vi "SPARK Configure Signal Period.vi"(8 "error in":errorcluster, 9 "Period (ms)":u32, 10 "Signal":T1, 11 "MotorControlDeviceRef":T2={"DeviceStatus"={"status"=FALSE, "code"=0, "source"=""}, "Type"=enum."PWM", "PWM"={"PWM Channel"=enum."Invalid", "DeadBand"={"Name"="", "maxPositivePwm"=0, "minPositivePwm"=0, "centerPwm"=0, "maxNegativePwm"=0, "minNegativePwm"=0, "angularRange"=0}}, "CAN"={"Device Number"=0, "SetOutput VI Ref"=variant(refnum<vi> refnum), "GetOutput VI Ref"=variant(refnum<vi> refnum), "Enable VI Ref"=variant(refnum<vi> refnum), "Disable VI Ref"=variant(refnum<vi> refnum), "Data"=variant}, "Invert"=FALSE, "DIO PWM"={"PWM \"Enable\" Channel"=enum."Invalid", "DIOChannel"=enum."Invalid", "PWM Rate"=0.0}}) -> (0 "error out":errorcluster, 3 "MotorControlDeviceRef":T2={"DeviceStatus"={"status"=FALSE, "code"=0, "source"=""}, "Type"=enum."PWM", "PWM"={"PWM Channel"=enum."Invalid", "DeadBand"={"Name"="", "maxPositivePwm"=0, "minPositivePwm"=0, "centerPwm"=0, "maxNegativePwm"=0, "minNegativePwm"=0, "angularRange"=0}}, "CAN"={"Device Number"=0, "SetOutput VI Ref"=variant(refnum<vi> refnum), "GetOutput VI Ref"=variant(refnum<vi> refnum), "Enable VI Ref"=variant(refnum<vi> refnum), "Disable VI Ref"=variant(refnum<vi> refnum), "Data"=variant}, "Invert"=FALSE, "DIO PWM"={"PWM \"Enable\" Channel"=enum."Invalid", "DIOChannel"=enum."Invalid", "PWM Rate"=0.0}})   [LabVIEW 2023]
doc: "Configure the period of a signal. This will be the rate at which the SPARK will send the periodic status that contains the specificed signal."
uses:
  <vilib>/Rock Robotics/WPI/MotorControl/WPI_MotorControlDeviceRef.ctl
  <vilib>/Rock Robotics/WPI/MotorControl/WPI_MotorControlType.ctl
  <vilib>/Rock Robotics/SystemInterfaces/DIO/FPGA_DIOPWMChannel.ctl
  <vilib>/Rock Robotics/WPI/PWM/WPI_PWMDeadband.ctl
  <vilib>/Rock Robotics/SystemInterfaces/DIO/FPGA_DIOChannel.ctl
  Typedef/SPARK Signal.ctl
  Typedef/SPARK Parameter ID.ctl
  Typedef/Spark MAX Variant Data.ctl
  Typedef/SPARK Model.ctl
  Private/SPARK/SPARK Set Parameter Uint32.vi
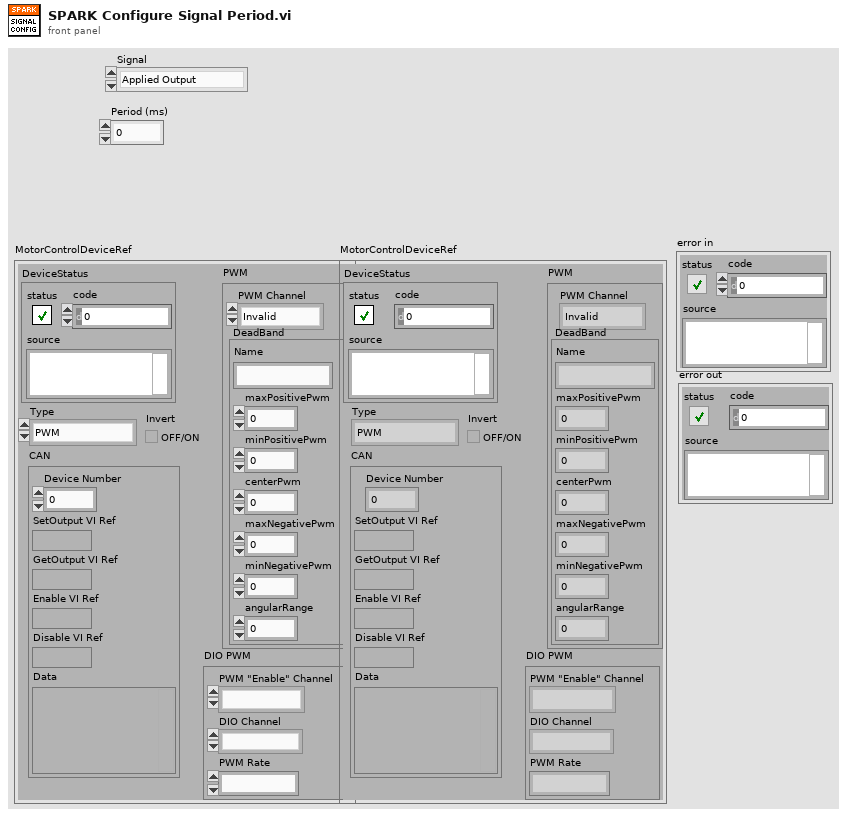
[diagram p1: front panel]
types:
  T1 = typedef "SPARK Signal.ctl" = enum16{"Applied Output", "Bus Voltage", "Output Current", "Motor Temperature", "Limits", "Faults", "Warnings", "Primary Encoder Velocity", "Primary Encoder Position", "Analog Voltage", "Analog Velocity", "Analog Position", "Alt/Ext Encoder Velocity", "Alt/Ext Encoder Position", "Absolute Encoder Velocity", "Absolute Encoder Position", "I Accumulation", "At Setpoint", "Setpoint", "Selected Closed Loop Slot", "MAXMotion Position Setpoint", "MAXMotion Velocity Setpoint"}
  T2 = typedef "WPI_MotorControlDeviceRef.ctl" = cluster{"DeviceStatus":errorcluster, "Type":T3, "PWM":cluster{"PWM Channel":T4, "DeadBand":T5}, "CAN":cluster{"Device Number":u8, "SetOutput VI Ref":variant, "GetOutput VI Ref":variant, "Enable VI Ref":variant, "Disable VI Ref":variant, "Data":variant}, "Invert":bool, "DIO PWM":cluster{"PWM \"Enable\" Channel":T4, "DIOChannel":T6, "PWM Rate":dbl}}
  T3 = typedef "WPI_MotorControlType.ctl" = enum16{"PWM", "CAN", "DIO PWM"}
  T4 = typedef "FPGA_DIOPWMChannel.ctl" = enum8{"PWM 0", "PWM 1", "PWM 2", "PWM 3", "PWM 4", "PWM 5", "PWM 6", "PWM 7", "PWM 8", "PWM 9", "PWM MXP 0", "PWM MXP 1", "PWM MXP 2", "PWM MXP 3", "PWM MXP 4", "PWM MXP 5", "PWM MXP 6", "PWM MXP 7", "PWM MXP 8", "PWM MXP 9", "Invalid"}
  T5 = typedef "WPI_PWMDeadband.ctl" = cluster{"Name":string, "maxPositivePwm":i32, "minPositivePwm":i32, "centerPwm":i32, "maxNegativePwm":i32, "minNegativePwm":i32, "angularRange":u16}
  T6 = typedef "FPGA_DIOChannel.ctl" = enum8{"DIO 0", "DIO 1", "DIO 2", "DIO 3", "DIO 4", "DIO 5", "DIO 6", "DIO 7", "DIO 8", "DIO 9", "DIO MXP 0", "DIO MXP 1", "DIO MXP 2", "DIO MXP 3", "DIO MXP 4", "DIO MXP 5", "DIO MXP 6", "DIO MXP 7", "DIO MXP 8", "DIO MXP 9", "DIO MXP 10", "DIO MXP 11", "DIO MXP 12", "DIO MXP 13", "DIO MXP 14", "DIO MXP 15", "SPI Port CS1", "SPI Port CS2", "SPI Port CS3", "SPI Port MISO", "SPI Port MOSI", "Invalid"}
  T7 = typedef "SPARK Parameter ID.ctl" = enum16{"kCanID", "kInputMode", "kMotorType", "kCommAdvance", "kSensorType", "kCtrlType", "kIdleMode", "kInputDeadband", "kLegacyFeedbackSensorPID0", "kClosedLoopControlSensor", "kPolePairs", "kCurrentChop", "kCurrentChopCycles", "kP_0", "kI_0", "kD_0", "kV_0", "kIZone_0", "kDFilter_0", "kOutputMin_0", "kOutputMax_0", "kP_1", "kI_1", "kD_1", "kV_1", "kIZone_1", "kDFilter_1", "kOutputMin_1", "kOutputMax_1", "kP_2", "kI_2", "kD_2", "kV_2", "kIZone_2", "kDFilter_2", "kOutputMin_2", "kOutputMax_2", "kP_3", "kI_3", "kD_3", "kV_3", "kIZone_3", "kDFilter_3", "kOutputMin_3", "kOutputMax_3", "kInverted", "kOutputRatio", "kSerialNumberLow", "kSerialNumberMid", "kSerialNumberHigh", "kLimitSwitchFwdPolarity", "kLimitSwitchRevPolarity", "kHardLimitFwdEn", "kHardLimitRevEn", "kSoftLimitFwdEn", "kSoftLimitRevEn", "kRampRate", "kFollowerID", "kFollowerConfig", "kSmartCurrentStallLimit", "kSmartCurrentFreeLimit", "kSmartCurrentConfig", "kSmartCurrentReserved", "kMotorKv", "kMotorR", "kMotorL", "kMotorRsvd1", "kMotorRsvd2", "kMotorRsvd3", "kEncoderCountsPerRev", "kEncoderAverageDepth", "kEncoderSampleDelta", "kEncoderInverted", "kEncoderRsvd1", "kClosedLoopVoltageMode", "kCompensatedNominalVoltage", "kSmartMotionMaxVelocity_0", "kSmartMotionMaxAccel_0", "kSmartMotionMinVelOutput_0", "kSmartMotionAllowedClosedLoopError_0", "kSmartMotionAccelStrategy_0", "kSmartMotionMaxVelocity_1", "kSmartMotionMaxAccel_1", "kSmartMotionMinVelOutput_1", "kSmartMotionAllowedClosedLoopError_1", "kSmartMotionAccelStrategy_1", "kSmartMotionMaxVelocity_2", "kSmartMotionMaxAccel_2", "kSmartMotionMinVelOutput_2", "kSmartMotionAllowedClosedLoopError_2", "kSmartMotionAccelStrategy_2", "kSmartMotionMaxVelocity_3", "kSmartMotionMaxAccel_3", "kSmartMotionMinVelOutput_3", "kSmartMotionAllowedClosedLoopError_3", "kSmartMotionAccelStrategy_3", "kIMaxAccum_0", "kAllowedClosedLoopError_0", "kSlot3Placeholder2_0", "kSlot3Placeholder3_0", "kIMaxAccum_1", "kAllowedClosedLoopError_1", "kSlot3Placeholder2_1", "kSlot3Placeholder3_1", "kIMaxAccum_2", "kAllowedClosedLoopError_2", "kSlot3Placeholder2_2", "kSlot3Placeholder3_2", "kIMaxAccum_3", "kAllowedClosedLoopError_3", "kSlot3Placeholder2_3", "kSlot3Placeholder3_3", "kPositionConversionFactor", "kVelocityConversionFactor", "kClosedLoopRampRate", "kSoftLimitFwd", "kSoftLimitRev", "kSoftLimitRsvd0", "kSoftLimitRsvd1", "kAnalogPositionConversion", "kAnalogVelocityConversion", "kAnalogAverageDepth", "kAnalogSensorMode", "kAnalogInverted", "kAnalogSampleDelta", "kAnalogRsvd0", "kAnalogRsvd1", "kDataPortConfig", "kAltEncoderCountsPerRev", "kAltEncoderAverageDepth", "kAltEncoderSampleDelta", "kAltEncoderInverted", "kAltEncoderPositionConversion", "kAltEncoderVelocityConversion", "kAltEncoderRsvd0", "kAltEncoderRsvd1", "kHallSensorSampleRate", "kHallSensorAverageDepth", "kNumParameters", "kDutyCyclePositionFactor", "kDutyCycleVelocityFactor", "kDutyCycleInverted", "kDutyCycleSensorMode", "kDutyCycleAverageDepth", "kDutyCycleSampleDelta", "kDutyCycleOffsetv1p6p2", "kDutyCycleRsvd0", "kDutyCycleRsvd1", "kDutyCycleRsvd2", "kPositionPIDWrapEnable", "kPositionPIDMinInput", "kPositionPIDMaxInput", "kDutyCycleZeroCentered", "kDutyCyclePrescalar", "kDutyCycleOffset", "kProductId", "kDeviceMajorVersion", "kDeviceMinorVersion", "kStatus0Period", "kStatus1Period", "kStatus2Period", "kStatus3Period", "kStatus4Period", "kStatus5Period", "kStatus6Period", "kStatus7Period", "kMAXMotionCruiseVelocity_0", "kMAXMotionMaxAccel_0", "kMAXMotionMaxJerk_0", "kMAXMotionAllowedProfileError_0", "kMAXMotionPositionMode_0", "kMAXMotionCruiseVelocity_1", "kMAXMotionMaxAccel_1", "kMAXMotionMaxJerk_1", "kMAXMotionAllowedProfileError_1", "kMAXMotionPositionMode_1", "kMAXMotionCruiseVelocity_2", "kMAXMotionMaxAccel_2", "kMAXMotionMaxJerk_2", "kMAXMotionAllowedProfileError_2", "kMAXMotionPositionMode_2", "kMAXMotionCruiseVelocity_3", "kMAXMotionMaxAccel_3", "kMAXMotionMaxJerk_3", "kMAXMotionAllowedProfileError_3", "kMAXMotionPositionMode_3", "kForceEnableStatus0", "kForceEnableStatus1", "kForceEnableStatus2", "kForceEnableStatus3", "kForceEnableStatus4", "kForceEnableStatus5", "kForceEnableStatus6", "kForceEnableStatus7", "kFollowerModeLeaderId", "kFollowerModeIsInverted", "kDutyCycleEncoderStartPulseUs", "kDutyCycleEncoderEndPulseUs", "kParamTableVersion", "kStatus8Period", "kForceEnableStatus8", "kLimitSwitchPositionSensor", "kLimitSwitchForwardPosition", "kLimitSwitchReversePosition", "kS_0", "kA_0", "kG_0", "kCos_0", "kCosRatio_0", "kS_1", "kA_1", "kG_1", "kCos_1", "kCosRatio_1", "kS_2", "kA_2", "kG_2", "kCos_2", "kCosRatio_2", "kS_3", "kA_3", "kG_3", "kCos_3", "kCosRatio_3", "kStatus9Period", "kForceEnableStatus9"}
  T8 = typedef "Spark MAX Variant Data.ctl" = cluster{"Ext ID":u32, "CAN Timeout":u32, "Inverted No WPILib":bool, "Has Configured Limit Sw":bool, "Has Configured Alt Encoder":bool, "SPARK Model":T9, "CAN Max Retries":u32, "CAN Timeout (ms)":u32, "Status 0 Period (ms)":u32, "Status 1 Period (ms)":u32, "Status 2 Period (ms)":u32, "Status 3 Period (ms)":u32, "Status 4 Period (ms)":u32, "Status 5 Period (ms)":u32, "Status 6 Period (ms)":u32, "Status 7 Period (ms)":u32, "Status 8 Period (ms)":u32, "Status 9 Period (ms)":u32, "Status Frame Timeout (ms)":u32}
  T9 = typedef "SPARK Model.ctl" = enum16{"SPARK MAX", "SPARK Flex", "Unknown"}
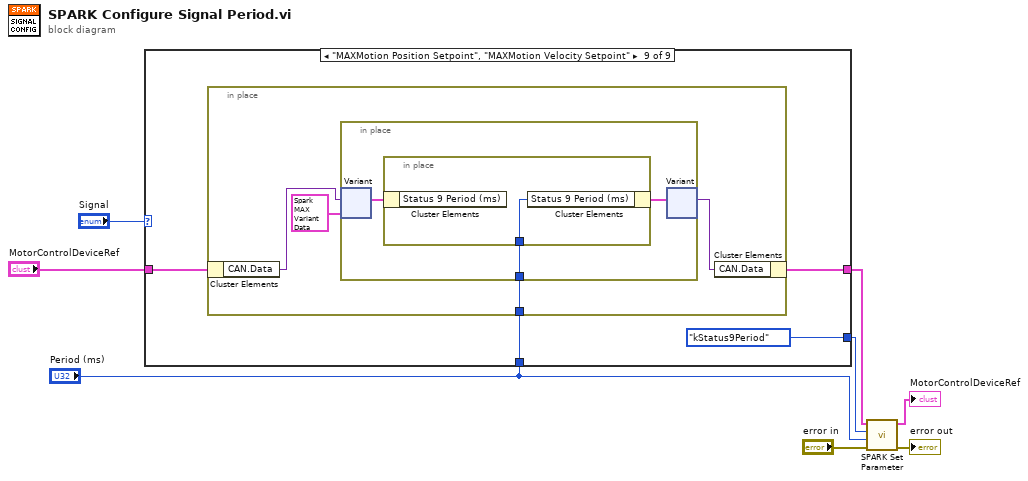
[diagram p0: block diagram]
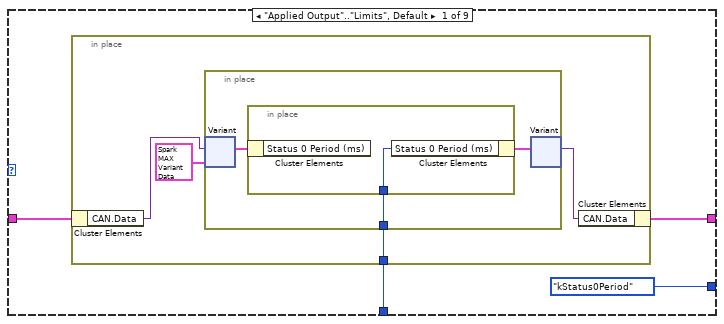
[diagram p2: hidden frame]
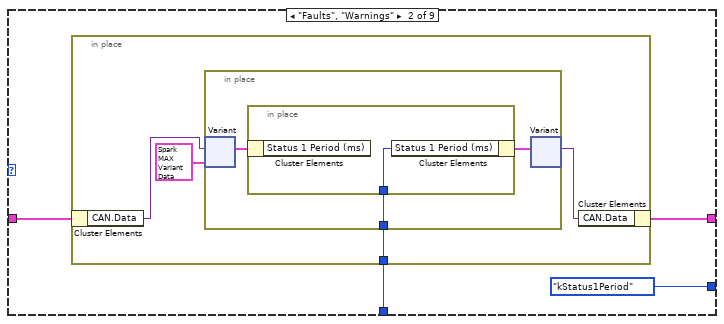
[diagram p3: hidden frame]
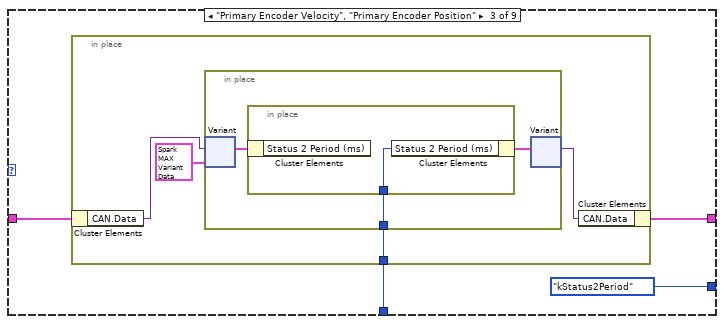
[diagram p4: hidden frame]
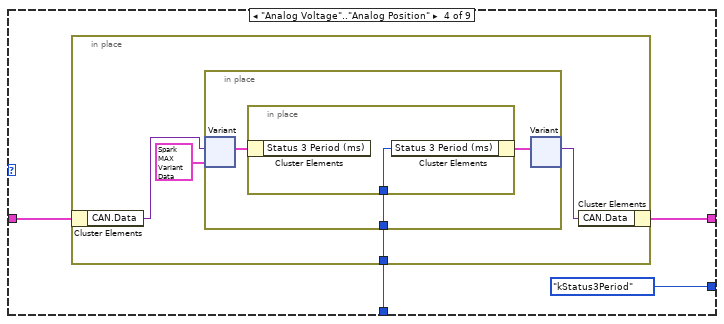
[diagram p5: hidden frame]
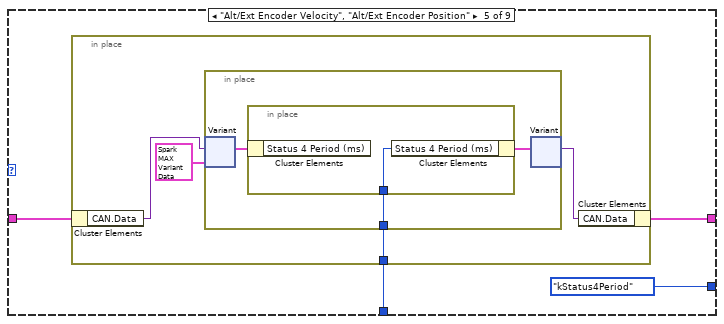
[diagram p6: hidden frame]
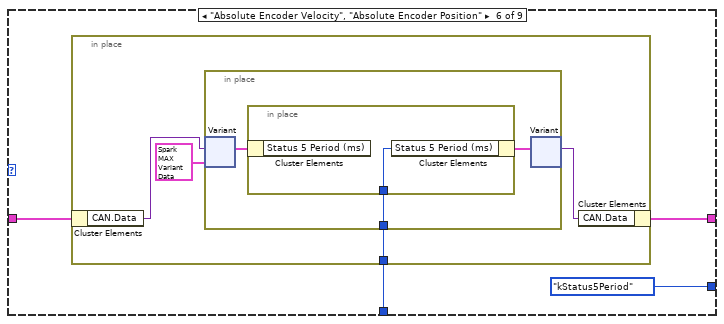
[diagram p7: hidden frame]
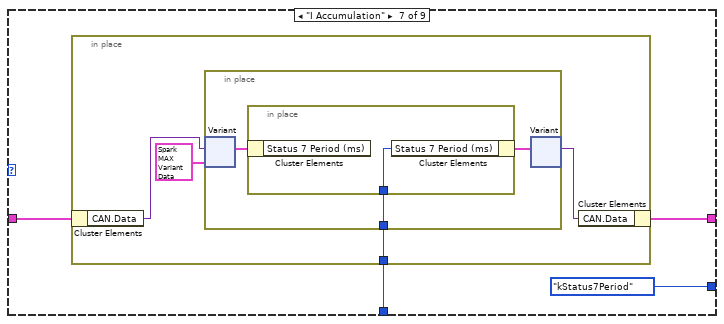
[diagram p8: hidden frame]
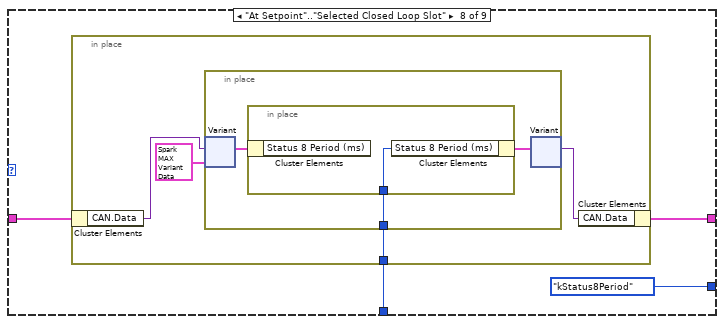
[diagram p9: hidden frame]
diagram:
  n1 = case shown="\"MAXMotion Position Setpoint\", \"MAXMotion Velocity Setpoint\"" "Signal" {
    tunnel: [SPARK_Parameter_ID."kStatus0Period" ("Parameter ID") SPARK_Parameter_ID."kStatus1Period" ("Parameter ID") SPARK_Parameter_ID."kStatus2Period" ("Parameter ID") SPARK_Parameter_ID."kStatus3Period" ("Parameter ID") SPARK_Parameter_ID."kStatus4Period" ("Parameter ID") SPARK_Parameter_ID."kStatus5Period" ("Parameter ID") SPARK_Parameter_ID."kStatus7Period" ("Parameter ID") SPARK_Parameter_ID."kStatus8Period" ("Parameter ID") SPARK_Parameter_ID."kStatus9Period" ("Parameter ID")] -> w7
    tunnel: "MotorControlDeviceRef" -> [w11 w22 w33 w46 w58 w70 w82 w94 w106]
    tunnel: "Period (ms)" -> [w10 w23 w35 w47 w59 w71 w83 w95 w107]
    tunnel: [w9 w21 w34 w45 w57 w69 w81 w93 w105] -> w1
    frame "Applied Output".."Limits", Default {
      n2 = in-place {
        in-place-border: w10 -> [w14]
        n3 = in-place-cluster #1(w11) -> ("CAN.Data"=w16:variant)
        n4 = in-place {
          in-place-border: w14 -> [w18]
          n5 = in-place-variant #2(w16, T8 {"Ext ID"=0, "CAN Timeout"=0, "Inverted No WPILib"=FALSE, "Has Configured Limit Sw"=FALSE, "Has Configured Alt Encoder"=FALSE, "SPARK Model"=enum."Unknown", "CAN Max Retries"=5, "CAN Timeout (ms)"=20, "Status 0 Period (ms)"=10, "Status 1 Period (ms)"=250, "Status 2 Period (ms)"=20, "Status 3 Period (ms)"=20, "Status 4 Period (ms)"=20, "Status 5 Period (ms)"=20, "Status 6 Period (ms)"=20, "Status 7 Period (ms)"=20, "Status 8 Period (ms)"=20, "Status 9 Period (ms)"=20, "Status Frame Timeout (ms)"=500} ("SPARK MAX Device Ref")) -> (w19:T8)  [unwired: 1 out]
          n6 = in-place {
            in-place-border: w18 -> [w20]
            n7 = in-place-cluster #3(w19) -> ()  [unwired: 1 out]
            n8 = in-place-cluster #3("Status 0 Period (ms)"=w20) -> (w17:T8)
          }
          n9 = in-place-variant #2(w17) -> (w13:variant)  [unwired: 1 out]
        }
        n10 = in-place-cluster #1("CAN.Data"=w13) -> (w9:T2)
      }
    }
    frame "Faults", "Warnings" {
      n11 = in-place {
        in-place-border: w23 -> [w26]
        n12 = in-place-cluster #4(w22) -> ("CAN.Data"=w28:variant)
        n13 = in-place {
          in-place-border: w26 -> [w30]
          n14 = in-place-variant #5(w28, T8 {"Ext ID"=0, "CAN Timeout"=0, "Inverted No WPILib"=FALSE, "Has Configured Limit Sw"=FALSE, "Has Configured Alt Encoder"=FALSE, "SPARK Model"=enum."Unknown", "CAN Max Retries"=5, "CAN Timeout (ms)"=20, "Status 0 Period (ms)"=10, "Status 1 Period (ms)"=250, "Status 2 Period (ms)"=20, "Status 3 Period (ms)"=20, "Status 4 Period (ms)"=20, "Status 5 Period (ms)"=20, "Status 6 Period (ms)"=20, "Status 7 Period (ms)"=20, "Status 8 Period (ms)"=20, "Status 9 Period (ms)"=20, "Status Frame Timeout (ms)"=500} ("SPARK MAX Device Ref")) -> (w31:T8)  [unwired: 1 out]
          n15 = in-place {
            in-place-border: w30 -> [w32]
            n16 = in-place-cluster #6(w31) -> ()  [unwired: 1 out]
            n17 = in-place-cluster #6("Status 1 Period (ms)"=w32) -> (w29:T8)
          }
          n18 = in-place-variant #5(w29) -> (w25:variant)  [unwired: 1 out]
        }
        n19 = in-place-cluster #4("CAN.Data"=w25) -> (w21:T2)
      }
    }
    frame "Primary Encoder Velocity", "Primary Encoder Position" {
      n20 = in-place {
        in-place-border: w35 -> [w38]
        n21 = in-place-cluster #7(w33) -> ("CAN.Data"=w40:variant)
        n22 = in-place {
          in-place-border: w38 -> [w42]
          n23 = in-place-variant #8(w40, T8 {"Ext ID"=0, "CAN Timeout"=0, "Inverted No WPILib"=FALSE, "Has Configured Limit Sw"=FALSE, "Has Configured Alt Encoder"=FALSE, "SPARK Model"=enum."Unknown", "CAN Max Retries"=5, "CAN Timeout (ms)"=20, "Status 0 Period (ms)"=10, "Status 1 Period (ms)"=250, "Status 2 Period (ms)"=20, "Status 3 Period (ms)"=20, "Status 4 Period (ms)"=20, "Status 5 Period (ms)"=20, "Status 6 Period (ms)"=20, "Status 7 Period (ms)"=20, "Status 8 Period (ms)"=20, "Status 9 Period (ms)"=20, "Status Frame Timeout (ms)"=500} ("SPARK MAX Device Ref")) -> (w43:T8)  [unwired: 1 out]
          n24 = in-place {
            in-place-border: w42 -> [w44]
            n25 = in-place-cluster #9(w43) -> ()  [unwired: 1 out]
            n26 = in-place-cluster #9("Status 2 Period (ms)"=w44) -> (w41:T8)
          }
          n27 = in-place-variant #8(w41) -> (w37:variant)  [unwired: 1 out]
        }
        n28 = in-place-cluster #7("CAN.Data"=w37) -> (w34:T2)
      }
    }
    frame "Analog Voltage".."Analog Position" {
      n29 = in-place {
        in-place-border: w47 -> [w50]
        n30 = in-place-cluster #10(w46) -> ("CAN.Data"=w52:variant)
        n31 = in-place {
          in-place-border: w50 -> [w54]
          n32 = in-place-variant #11(w52, T8 {"Ext ID"=0, "CAN Timeout"=0, "Inverted No WPILib"=FALSE, "Has Configured Limit Sw"=FALSE, "Has Configured Alt Encoder"=FALSE, "SPARK Model"=enum."Unknown", "CAN Max Retries"=5, "CAN Timeout (ms)"=20, "Status 0 Period (ms)"=10, "Status 1 Period (ms)"=250, "Status 2 Period (ms)"=20, "Status 3 Period (ms)"=20, "Status 4 Period (ms)"=20, "Status 5 Period (ms)"=20, "Status 6 Period (ms)"=20, "Status 7 Period (ms)"=20, "Status 8 Period (ms)"=20, "Status 9 Period (ms)"=20, "Status Frame Timeout (ms)"=500} ("SPARK MAX Device Ref")) -> (w55:T8)  [unwired: 1 out]
          n33 = in-place {
            in-place-border: w54 -> [w56]
            n34 = in-place-cluster #12(w55) -> ()  [unwired: 1 out]
            n35 = in-place-cluster #12("Status 3 Period (ms)"=w56) -> (w53:T8)
          }
          n36 = in-place-variant #11(w53) -> (w49:variant)  [unwired: 1 out]
        }
        n37 = in-place-cluster #10("CAN.Data"=w49) -> (w45:T2)
      }
    }
    frame "Alt/Ext Encoder Velocity", "Alt/Ext Encoder Position" {
      n38 = in-place {
        in-place-border: w59 -> [w62]
        n39 = in-place-cluster #13(w58) -> ("CAN.Data"=w64:variant)
        n40 = in-place {
          in-place-border: w62 -> [w66]
          n41 = in-place-variant #14(w64, T8 {"Ext ID"=0, "CAN Timeout"=0, "Inverted No WPILib"=FALSE, "Has Configured Limit Sw"=FALSE, "Has Configured Alt Encoder"=FALSE, "SPARK Model"=enum."Unknown", "CAN Max Retries"=5, "CAN Timeout (ms)"=20, "Status 0 Period (ms)"=10, "Status 1 Period (ms)"=250, "Status 2 Period (ms)"=20, "Status 3 Period (ms)"=20, "Status 4 Period (ms)"=20, "Status 5 Period (ms)"=20, "Status 6 Period (ms)"=20, "Status 7 Period (ms)"=20, "Status 8 Period (ms)"=20, "Status 9 Period (ms)"=20, "Status Frame Timeout (ms)"=500} ("SPARK MAX Device Ref")) -> (w67:T8)  [unwired: 1 out]
          n42 = in-place {
            in-place-border: w66 -> [w68]
            n43 = in-place-cluster #15(w67) -> ()  [unwired: 1 out]
            n44 = in-place-cluster #15("Status 4 Period (ms)"=w68) -> (w65:T8)
          }
          n45 = in-place-variant #14(w65) -> (w61:variant)  [unwired: 1 out]
        }
        n46 = in-place-cluster #13("CAN.Data"=w61) -> (w57:T2)
      }
    }
    frame "Absolute Encoder Velocity", "Absolute Encoder Position" {
      n47 = in-place {
        in-place-border: w71 -> [w74]
        n48 = in-place-cluster #16(w70) -> ("CAN.Data"=w76:variant)
        n49 = in-place {
          in-place-border: w74 -> [w78]
          n50 = in-place-variant #17(w76, T8 {"Ext ID"=0, "CAN Timeout"=0, "Inverted No WPILib"=FALSE, "Has Configured Limit Sw"=FALSE, "Has Configured Alt Encoder"=FALSE, "SPARK Model"=enum."Unknown", "CAN Max Retries"=5, "CAN Timeout (ms)"=20, "Status 0 Period (ms)"=10, "Status 1 Period (ms)"=250, "Status 2 Period (ms)"=20, "Status 3 Period (ms)"=20, "Status 4 Period (ms)"=20, "Status 5 Period (ms)"=20, "Status 6 Period (ms)"=20, "Status 7 Period (ms)"=20, "Status 8 Period (ms)"=20, "Status 9 Period (ms)"=20, "Status Frame Timeout (ms)"=500} ("SPARK MAX Device Ref")) -> (w79:T8)  [unwired: 1 out]
          n51 = in-place {
            in-place-border: w78 -> [w80]
            n52 = in-place-cluster #18(w79) -> ()  [unwired: 1 out]
            n53 = in-place-cluster #18("Status 5 Period (ms)"=w80) -> (w77:T8)
          }
          n54 = in-place-variant #17(w77) -> (w73:variant)  [unwired: 1 out]
        }
        n55 = in-place-cluster #16("CAN.Data"=w73) -> (w69:T2)
      }
    }
    frame "I Accumulation" {
      n56 = in-place {
        in-place-border: w83 -> [w86]
        n57 = in-place-cluster #19(w82) -> ("CAN.Data"=w88:variant)
        n58 = in-place {
          in-place-border: w86 -> [w90]
          n59 = in-place-variant #20(w88, T8 {"Ext ID"=0, "CAN Timeout"=0, "Inverted No WPILib"=FALSE, "Has Configured Limit Sw"=FALSE, "Has Configured Alt Encoder"=FALSE, "SPARK Model"=enum."Unknown", "CAN Max Retries"=5, "CAN Timeout (ms)"=20, "Status 0 Period (ms)"=10, "Status 1 Period (ms)"=250, "Status 2 Period (ms)"=20, "Status 3 Period (ms)"=20, "Status 4 Period (ms)"=20, "Status 5 Period (ms)"=20, "Status 6 Period (ms)"=20, "Status 7 Period (ms)"=20, "Status 8 Period (ms)"=20, "Status 9 Period (ms)"=20, "Status Frame Timeout (ms)"=500} ("SPARK MAX Device Ref")) -> (w91:T8)  [unwired: 1 out]
          n60 = in-place {
            in-place-border: w90 -> [w92]
            n61 = in-place-cluster #21(w91) -> ()  [unwired: 1 out]
            n62 = in-place-cluster #21("Status 7 Period (ms)"=w92) -> (w89:T8)
          }
          n63 = in-place-variant #20(w89) -> (w85:variant)  [unwired: 1 out]
        }
        n64 = in-place-cluster #19("CAN.Data"=w85) -> (w81:T2)
      }
    }
    frame "At Setpoint".."Selected Closed Loop Slot" {
      n65 = in-place {
        in-place-border: w95 -> [w98]
        n66 = in-place-cluster #22(w94) -> ("CAN.Data"=w100:variant)
        n67 = in-place {
          in-place-border: w98 -> [w102]
          n68 = in-place-variant #23(w100, T8 {"Ext ID"=0, "CAN Timeout"=0, "Inverted No WPILib"=FALSE, "Has Configured Limit Sw"=FALSE, "Has Configured Alt Encoder"=FALSE, "SPARK Model"=enum."Unknown", "CAN Max Retries"=5, "CAN Timeout (ms)"=20, "Status 0 Period (ms)"=10, "Status 1 Period (ms)"=250, "Status 2 Period (ms)"=20, "Status 3 Period (ms)"=20, "Status 4 Period (ms)"=20, "Status 5 Period (ms)"=20, "Status 6 Period (ms)"=20, "Status 7 Period (ms)"=20, "Status 8 Period (ms)"=20, "Status 9 Period (ms)"=20, "Status Frame Timeout (ms)"=500} ("SPARK MAX Device Ref")) -> (w103:T8)  [unwired: 1 out]
          n69 = in-place {
            in-place-border: w102 -> [w104]
            n70 = in-place-cluster #24(w103) -> ()  [unwired: 1 out]
            n71 = in-place-cluster #24("Status 8 Period (ms)"=w104) -> (w101:T8)
          }
          n72 = in-place-variant #23(w101) -> (w97:variant)  [unwired: 1 out]
        }
        n73 = in-place-cluster #22("CAN.Data"=w97) -> (w93:T2)
      }
    }
    frame "MAXMotion Position Setpoint", "MAXMotion Velocity Setpoint" {
      n74 = in-place {
        in-place-border: w107 -> [w110]
        n75 = in-place-cluster #25(w106) -> ("CAN.Data"=w112:variant)
        n76 = in-place {
          in-place-border: w110 -> [w114]
          n77 = in-place-variant #26(w112, T8 {"Ext ID"=0, "CAN Timeout"=0, "Inverted No WPILib"=FALSE, "Has Configured Limit Sw"=FALSE, "Has Configured Alt Encoder"=FALSE, "SPARK Model"=enum."Unknown", "CAN Max Retries"=5, "CAN Timeout (ms)"=20, "Status 0 Period (ms)"=10, "Status 1 Period (ms)"=250, "Status 2 Period (ms)"=20, "Status 3 Period (ms)"=20, "Status 4 Period (ms)"=20, "Status 5 Period (ms)"=20, "Status 6 Period (ms)"=20, "Status 7 Period (ms)"=20, "Status 8 Period (ms)"=20, "Status 9 Period (ms)"=20, "Status Frame Timeout (ms)"=500} ("SPARK MAX Device Ref")) -> (w115:T8)  [unwired: 1 out]
          n78 = in-place {
            in-place-border: w114 -> [w116]
            n79 = in-place-cluster #27(w115) -> ()  [unwired: 1 out]
            n80 = in-place-cluster #27("Status 9 Period (ms)"=w116) -> (w113:T8)
          }
          n81 = in-place-variant #26(w113) -> (w109:variant)  [unwired: 1 out]
        }
        n82 = in-place-cluster #25("CAN.Data"=w109) -> (w105:T2)
      }
    }
  }
  n83 = call-poly "SPARK Set Parameter.vi"("error in (no error)"="error in", "uint"="Period (ms)", "Parameter ID"=w7, "MotorControlDeviceRef"=w1) -> ("error out"=→"error out":errorcluster, "MotorControlDeviceRef"=→"MotorControlDeviceRef":T2)  [unwired: 6 in]
